vi "Add Status Section.vi"(8 "error in":errorcluster, 11 "custom device ref":T1 format="%.0x") -> (0 "error out":errorcluster, 2 "status ref":T1 format="%.0x", 3 "custom device ref out":T1 format="%.0x")   [LabVIEW 2020, in "Ballard ARINC 429 Scripting.lvlib"]
uses:
  Ballard ARINC 429 Scripting.lvlib
  <vilib>/NI VeriStand/Custom Device API/Custom Device Item Ref.ctl
  Constants.vi
  <vilib>/NI VeriStand/Custom Device Offline API/Custom Device Offline API.lvlib
  <vilib>/NI VeriStand/Custom Device API/Custom Device API.lvlib
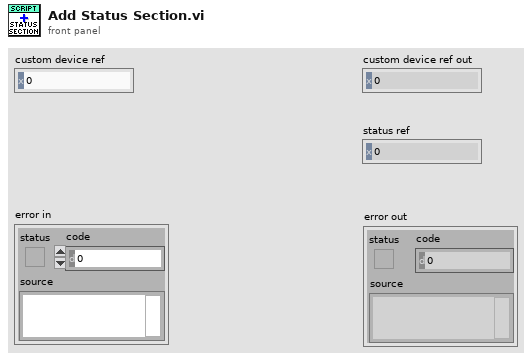
[diagram p1: front panel]
types:
  T1 = typedef "Custom Device API.lvlib/Custom Device Item Ref.ctl" = u64
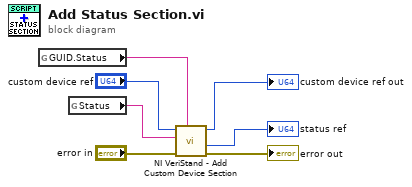
[diagram p0: block diagram]
diagram:
  n1 = global read "Constants.vi" "GUID.Status"() -> (w1:string)
  n2 = global read "Constants.vi" "Status"() -> (w2:string)
  n3 = call <vilib>:"NI VeriStand - Add Custom Device Section.vi"("GUID (Default Section)"=w1, "error in (no error)"="error in", "Section Name"=w2, "Parent Ref in"="custom device ref") -> ("error out"=→"error out":errorcluster, "Section Ptr"=→"status ref":T1, "Parent Ref out"=→"custom device ref out":T1)  [unwired: 4 in, 1 out]
